vi "Init SPI CS.vi"(8 "error in (no error)":errorcluster, 10 "SPI CS In":refnum<class "SPI CS.lvclass">, 11 "Session in":refnum<class "Session.lvclass">) -> (0 "error out":errorcluster, 2 "SPI CS":refnum<class "SPI CS.lvclass">, 3 "Session out":refnum<class "Session.lvclass">)   [LabVIEW 2024, in "CTI.lvlib" / "Session.lvclass"]
uses:
  Session.lvclass
  SPI CS/SPI CS.lvclass
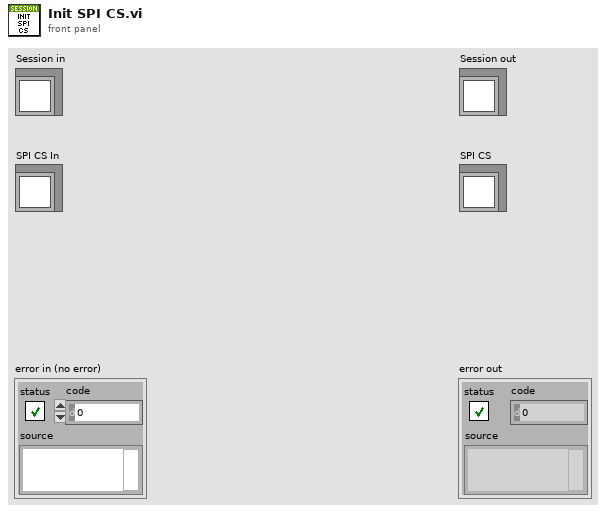
[diagram p1: front panel]
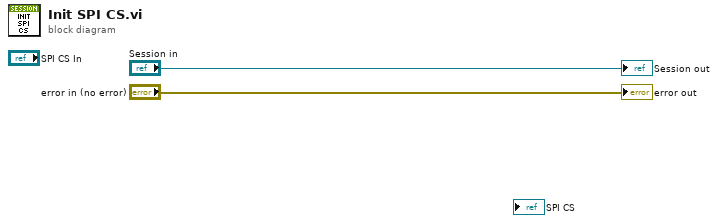
[diagram p0: block diagram]
diagram:
  "error out" <- "error in (no error)"
  "Session out" <- "Session in"
